vi "server.vi"(8 "error in (no error)":errorcluster, 9 "Origin":T1, 10 "Window Dimensions":cluster{"width":i16, "height":i16}, 11 "path in":path) -> (0 "error out":errorcluster, 3 "path out":path)   [LabVIEW 2016]
uses:
  <vilib>/Utility/miscctls.llb/LVPointTypeDef.ctl
  <vilib>/Utility/miscctls.llb/LVRectTypeDef.ctl
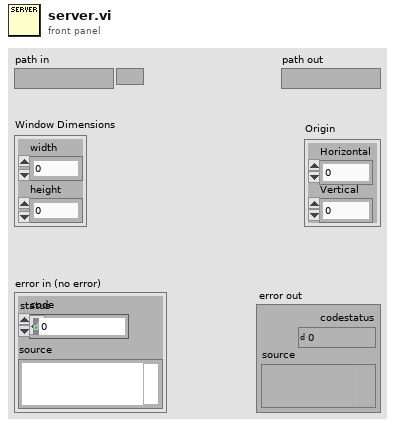
[diagram p1: front panel]
types:
  T1 = typedef "LVPointTypeDef.ctl" = cluster{"Horizontal":i16, "Vertical":i16}
  T2 = typedef "LVRectTypeDef.ctl" = cluster{"Left":i16, "Top":i16, "Right":i16, "Bottom":i16}
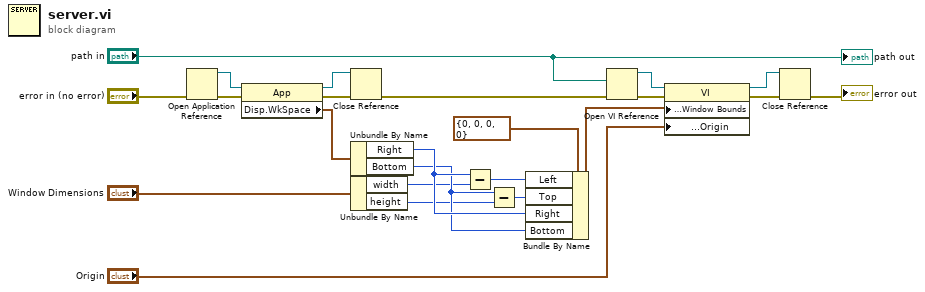
[diagram p0: block diagram]
diagram:
  n1 = Open Application Reference(8:"error in (no error)") -> (0:w20:errorcluster, 3:w22:refnum<vi>)  [unwired: 3 out]
  n2 = property class="App"(reference=w22, error in=w20) -> (reference out=w21:refnum<vi>, error out=w19:errorcluster, "Disp.WkSpace"=w17:T2)
  n3 = Close Reference(reference=w21, error in (no error)=w19) -> (error out=w18:errorcluster)
  n4 = Unbundle By Name(w17) -> ("Right"=w16:i16, "Bottom"=w14:i16)
  n5 = Unbundle By Name("Window Dimensions") -> ("width"=w11:i16, "height"=w10:i16)
  n6 = Subtract(x=w16, y=w11) -> (x-y=w15:i16)
  n7 = Subtract(x=w14, y=w10) -> (x-y=w13:i16)
  n8 = Bundle By Name(cluster=T2 {"Left"=0, "Top"=0, "Right"=0, "Bottom"=0} ("Front Panel Window:Window Bounds"), "Left"=w15, "Top"=w13, "Right"=w16, "Bottom"=w14) -> (w5:T2)
  n9 = Open VI Reference(vi path="path in", error in (no error)=w18) -> (vi reference=w8:refnum<vi>, error out=w7:errorcluster)  [unwired: 4 out]
  n10 = property class="VI"(reference=w8, error in=w7, "Front Panel Window:Window Bounds"=w5, "Front Panel Window:Origin"="Origin") -> (reference out=w6:refnum<vi>, error out=w3:errorcluster)
  n11 = Close Reference(reference=w6, error in (no error)=w3) -> (error out=→"error out":errorcluster)
  "path out" <- "path in"
